vi "png path to tdms image path.vi"(8 "error in (no error)":errorcluster, 11 "png path":path) -> (0 "error out":errorcluster, 1 "tdms index path":path, 2 "Dev name":string, 3 "tdms image path":path)   [LabVIEW 2020]
panel:
  out "ScanFolderName":string
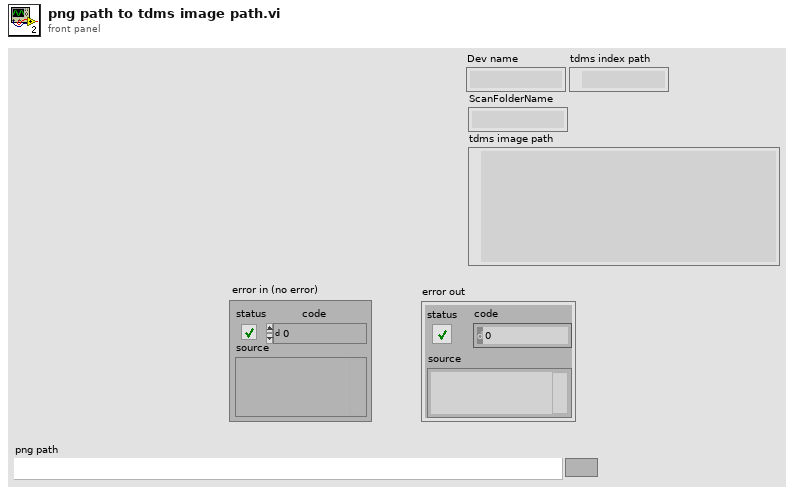
[diagram p1: front panel]
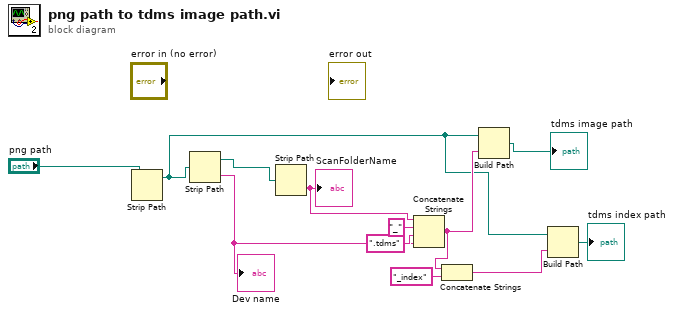
[diagram p0: block diagram]
diagram:
  n1 = Strip Path(path="png path") -> (stripped path=w3:path)  [unwired: 1 out]
  n2 = Strip Path(path=w3) -> (stripped path=w12:path, name=w9:string)
  "Dev name" <- w9
  n3 = Strip Path(path=w12) -> (name=w10:string)  [unwired: 1 out]
  "ScanFolderName" <- w10
  n4 = Concatenate Strings(w10, "_" ("string"), w9, ".tdms" ("string")) -> (w5:string)
  n5 = Concatenate Strings(w5, "_index" ("string")) -> (w2:string)
  n6 = Build Path(base path=w3, name or relative path=w5) -> (appended path=→"tdms image path":path)
  n7 = Build Path(base path=w3, name or relative path=w2) -> (appended path=→"tdms index path":path)
